vi "Find Workspace.vi"(6 "Pickup_Test_Number":dbl, 8 "Error In":errorcluster, 9 "Assembly Type":string, 10 "Control In":T2={"I-O.lvclass"=refnum, "Gantry"=refnum, "Dispenser"="COM1"}, 11 "Workspace In":refnum<class "Fixture.lvclass">) -> (0 "Error Out":errorcluster, 1 "Workspace Out":T1, 2 "Control Out":T2={"I-O.lvclass"=refnum, "Gantry"=refnum, "Dispenser"="COM1"}, 3 "Workspace Out":refnum<class "Fixture.lvclass">)   [LabVIEW 2021, in "Fixture.lvclass"]
uses:
  Fixture.lvclass
  Controller/Controllers.ctl
  Controller/I-O/I-O.lvclass
  C:/Program Files (x86)/Aerotech/A3200/LabVIEW/2010/Bin/Aerotech.A3200.dll
  Program Files (x86)/Aerotech/A3200/LabVIEW/2010/Bin/Aerotech.A3200.dll
  Workspace.ctl
  Fixture.lvclass/Fixture.ctl
  Controller/Controller.lvclass
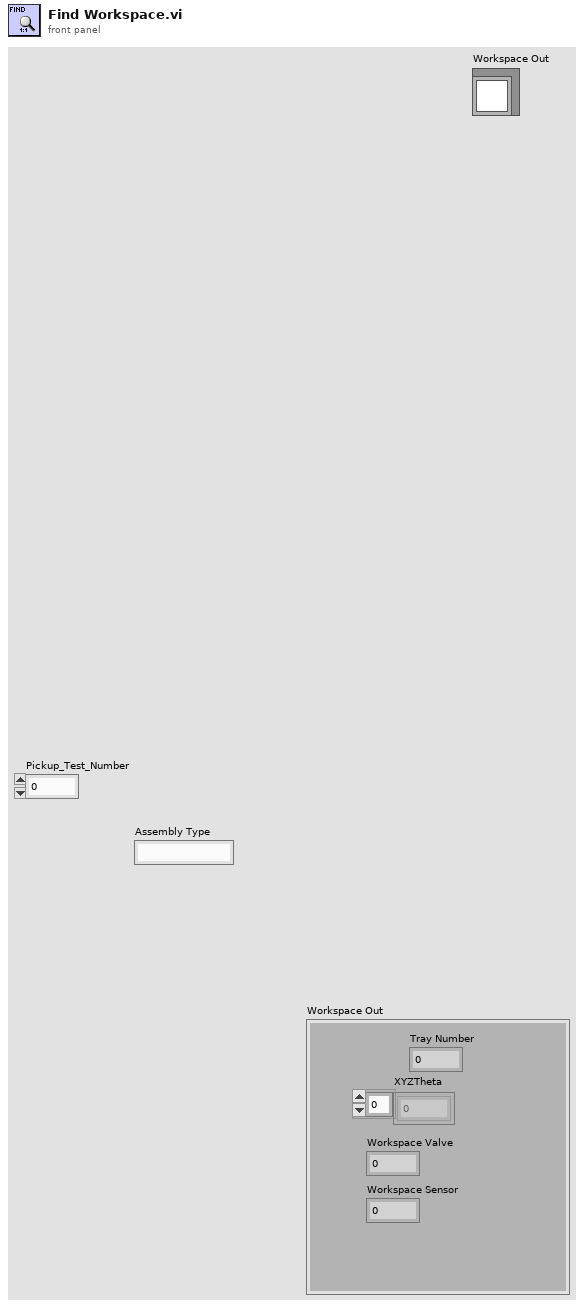
[diagram p1: front panel]
types:
  T1 = typedef "Fixture.lvclass/Workspace.ctl" = cluster{"XYZTheta":dbl[], "Workspace Valve":i32, "Workspace Sensor":i32, "Tray Number":i32}
  T2 = typedef "Controller.lvclass/Controllers.ctl" = cluster{"I-O.lvclass":refnum<class "I-O.lvclass">, "Gantry":refnum<k24>, "Dispenser":refnum<visa-resource-name>}
  T3 = typedef "I-O.lvclass/Pin Map.ctl" = cluster{"Region Valves":i32[], "Extra Valves":dbl[][][], "Tool Primary Valve":i32, "Tool Secondary Valve":i32, "Region Sensors":i32[], "Extra Sensors":dbl[][][], "Tool Primary Sensor":dbl, "Tool Secondary Sensor":dbl, "Compression Sensor":dbl, "5V":i32, "Dispenser Sensor":dbl}
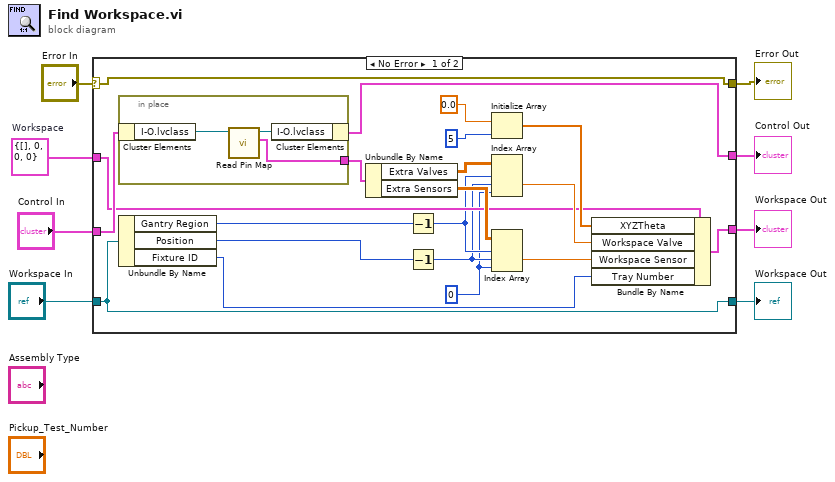
[diagram p0: block diagram]
diagram:
  w4 = T1 {"XYZTheta"=[], "Workspace Valve"=0, "Workspace Sensor"=0, "Tray Number"=0}  # Workspace
  n1 = case shown="No Error" "Error In" {
    selector: "Error In" -> [w28 w35]
    tunnel: [w28 w35] -> w7
    tunnel: [w23 w34] -> w5
    tunnel: "Workspace In" -> [w23 w34]
    tunnel: w4 -> [w15 w33]
    tunnel: [w17 w33] -> w3
    tunnel: "Control In" -> [w27 w32]
    tunnel: [w26 w32] -> w1
    frame No Error {
      w10 = 0
      n2 = in-place {
        in-place-border: [w29] -> w22
        n3 = in-place-cluster #1(w27) -> ("I-O.lvclass"=w31:refnum<class "I-O.lvclass">)
        n4 = call-dynamic "Read Pin Map.vi"("I-O in"=w31) -> ("Pin Map 2"=w29:T3, "I-O out"=w30:refnum<class "I-O.lvclass">)  [unwired: 8 in, 1 out]
        n5 = in-place-cluster #1("I-O.lvclass"=w30) -> (w26:T2)
      }
      n6 = Unbundle By Name(w23) -> ("Gantry Region"=w14:i32, "Position"=w12:i32, "Fixture ID"=w9:i32)
      n7 = Unbundle By Name(w22) -> ("Extra Valves"=w21:dbl[][][], "Extra Sensors"=w20:dbl[][][])
      n8 = Decrement(x=w14) -> (x-1=w13:i32)
      n9 = Decrement(x=w12) -> (x-1=w11:i32)
      n10 = Initialize Array "Initialize Array"(0.0 ("element"), 5 ("dimension size")) -> (w16:dbl[])
      n11 = Index Array(array=w21, index (dim 0)=w13, index (dim 1)=w11, index (dim 2)=w10) -> (element=w19:dbl)
      n12 = Index Array "Index Array"(array=w20, index (dim 0)=w13, index (dim 1)=w11, index (dim 2)=w10) -> (element=w18:dbl)
      n13 = Bundle By Name(cluster=w15, "XYZTheta"=w16, "Workspace Valve"=w19, "Workspace Sensor"=w18, "Tray Number"=w9) -> (w17:T1)
    }
    frame Error {
    }
  }
  "Error Out" <- w7
  "Workspace Out" <- w5
  "Control Out" <- w1
  "Workspace Out" <- w3
